vi "PDU Close.vi"(8 "error in (no error)":errorcluster, 11 "Orion PDU in":refnum<class "Orion PDU.lvclass">) -> (0 "error out":errorcluster, 3 "Orion PDU out":refnum<class "Orion PDU.lvclass">)   [LabVIEW 2022 SP3, in "Orion PDU.lvclass"]
uses:
  Orion PDU.lvclass
  Orion PDU.lvclass/Orion PDU.ctl
  Power Distribution.lvclass
  <vilib>/httpClient/LabVIEWHTTPClient.lvlib
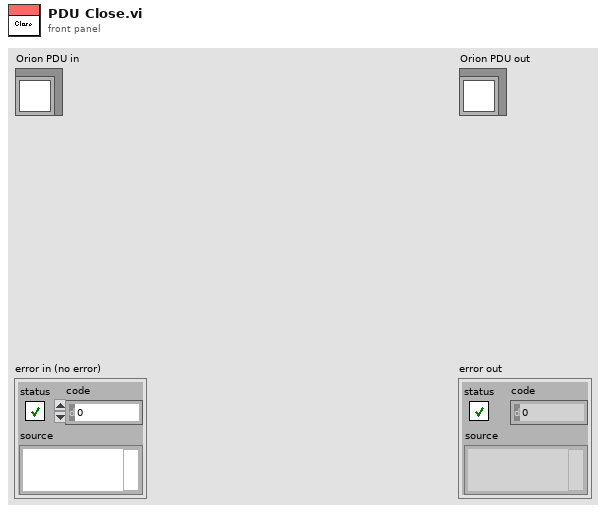
[diagram p1: front panel]
types:
  T1 = typedef "LabVIEWHTTPClient.lvlib/ClientHandle.ctl" = refnum<k1>
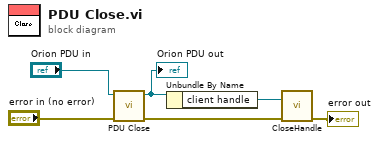
[diagram p0: block diagram]
diagram:
  n1 = call-parent "PDU Close.vi"("error in (no error)"="error in (no error)", "Power Distribution in"="Orion PDU in") -> ("error out"=w2:errorcluster, "Power Distribution out"=w4:refnum<class "Orion PDU.lvclass">)  [unwired: 8 in]
  "Orion PDU out" <- w4
  n2 = Unbundle By Name(w4) -> ("client handle"=w3:T1)
  n3 = call <vilib>:"CloseHandle.vi"("client handle"=w3, "error in (no error)"=w2) -> ("error out"=→"error out":errorcluster)  [unwired: 13 in]
